vi "写入excel(参考灵敏度).vi"(7 "设置":string[](array[string])=["160", "10", "0.02", "0.02", "0.1", "10", "J5", "J6"], 8 "error in (no error)":errorcluster, 9 "被测幅值":dbl[](array[numeric]), 10 "参考幅值":dbl format="%.2p", 11 "NI_report输入":refnum<class "NI_report.lvclass">) -> (0 "error out":errorcluster, 3 "report out":refnum<class "NI_report.lvclass">)   [LabVIEW 2015]
uses:
  <vilib>/Utility/NIReport.llb/NI_report.lvclass
  <vilib>/addons/_office/_exclsub.llb/font.ctl
  Global.vi
  <vilib>/Utility/NIReport.llb/Excel/NI_Excel.lvclass
  <vilib>/addons/_office/NI_ReportGenerationToolkit.lvlib
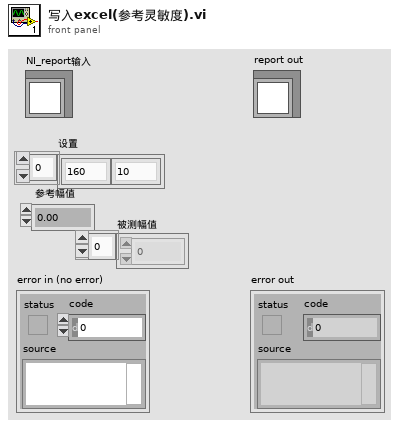
[diagram p1: front panel]
types:
  T1 = typedef "NI_ReportGenerationToolkit.lvlib/font.ctl" = cluster{"font name":string, "font size":dbl, "bold":u16, "italic":u16, "underline":u16, "strike through":u16, "font color":u32}
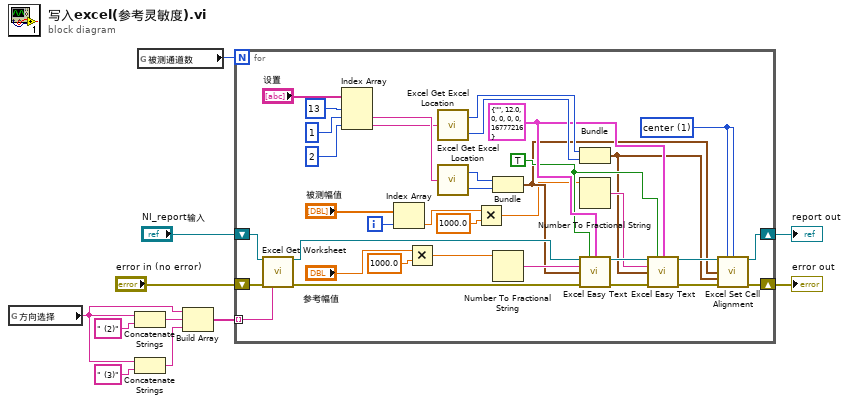
[diagram p0: block diagram]
diagram:
  n1 = global read "Global.vi" "方向选择"() -> (w5:string)
  n2 = Concatenate Strings(w5, " (2)") -> (w4:string)
  n3 = Concatenate Strings(w5, " (3)") -> (w3:string)
  n4 = global read "Global.vi" "被测通道数"() -> (w1:i32)
  n5 = Build Array(w5, w4, w3) -> (w2:string[])
  n6 = for {
    N: w1 -> [_]
    shift-right: [w25] -> w9
    shift-left: "NI_report输入" -> [w47]
    shift-right: [w24] -> w8
    shift-left: "error in (no error)" -> [w46]
    tunnel: w2 -> [w15] mode=indexing
    i -> [w13]
    w21 = 1 items=["top", "center", "bottom"] ("vertical alignment (top)")
    w28 = TRUE ("border? (F)")
    w29 = T1 {"font name"="", "font size"=12.0, "bold"=0, "italic"=0, "underline"=0, "strike through"=0, "font color"=16777216} ("font")
    n7 = call <vilib>:"Excel Get Worksheet.vi"("report in"=w47, "error in (no error)"=w46, "name (\"\")"=w15) -> ("report out"=w45:refnum<class "NI_report.lvclass">, "error out"=w44:errorcluster)  [unwired: 11 in]
    n8 = Index Array(array="设置", index #1=13 ("索引"), index #2=1 ("索引 (行)"), index #3=2 ("索引")) -> (element #2=w38:string, element #3=w32:string)  [unwired: 1 out]
    n9 = Index Array(array="被测幅值", index=w13) -> (element=w12:dbl)
    n10 = Multiply(x="参考幅值", y=1000.0) -> (x*y=w16:dbl)
    n11 = call <vilib>:"Excel Get Excel Location.vi"("cell's name"=w32) -> ("row"=w31:i32, "column"=w30:i32)
    n12 = call <vilib>:"Excel Get Excel Location.vi"("cell's name"=w38) -> ("row"=w37:i32, "column"=w36:i32)
    n13 = Multiply(x=w12, y=1000.0) -> (x*y=w19:dbl)
    n14 = Bundle("row"=w37, "column"=w36) -> (w23:cluster{"row":i32, "column":i32})  [unwired: 1 in]
    n15 = Number To Fractional String(number=w16) -> (F-format string=w39:string)  [unwired: 3 in]
    n16 = Bundle("row"=w31, "column"=w30) -> (w22:cluster{"row":i32, "column":i32})  [unwired: 1 in]
    n17 = Number To Fractional String(number=w19) -> (F-format string=w33:string)  [unwired: 3 in]
    n18 = call <vilib>:"Excel Easy Text.vi"("report in"=w45, "border? (F)"=w28, "font"=w29, "text"=w39, "start (-1, -1)"=w23, "error in (no error)"=w44) -> ("report out"=w35:refnum<class "NI_report.lvclass">, "error out"=w34:errorcluster)  [unwired: 5 in, 3 out]
    n19 = call <vilib>:"Excel Easy Text.vi"("report in"=w35, "border? (F)"=w28, "font"=w29, "text"=w33, "start (-1, -1)"=w22, "error in (no error)"=w34) -> ("report out"=w27:refnum<class "NI_report.lvclass">, "error out"=w26:errorcluster)  [unwired: 5 in, 3 out]
    n20 = call <vilib>:"Excel Set Cell Alignment.vi"("report in"=w27, "vertical alignment (top)"=w21, "horizontal alignment (left)"=w21, "start (-1, -1)"=w23, "end (-1, -1)"=w22, "error in (no error)"=w26) -> ("report out"=w25:refnum<class "NI_report.lvclass">, "error out"=w24:errorcluster)  [unwired: 8 in]
  }
  "report out" <- w9
  "error out" <- w8
